vi "getState.vi"(8 "error in (no error)":errorcluster, 11 "UntilIntensityReading in":refnum<class "UntilIntensityReading.lvclass">) -> (0 "error out":errorcluster, 2 "StateValue":T1=enum."UntilIntensityReadingState", 3 "UntilIntensityReading out":refnum<class "UntilIntensityReading.lvclass">)   [LabVIEW 2016, in "UntilIntensityReading.lvclass"]
uses:
  UntilIntensityReading.lvclass
  ts_electrometeruserevents/Typedefs/StateValue.ctl
  ts_electrometeruserevents/Typedefs/ElectrometerTypedefs.lvlib
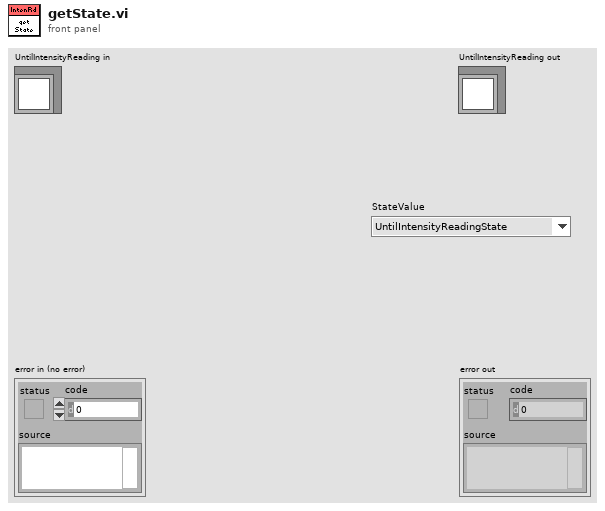
[diagram p1: front panel]
types:
  T1 = typedef "ElectrometerTypedefs.lvlib/StateValue.ctl" = enum16{"", "DisabledState", "EnabledState", "FaultState", "OffState", "StandbyState", "ReadyState", "ConfiguringState", "ManualReadingState", "UntilIntensityReadingState", "SetDurationReadingState", "BufferReadingState"}
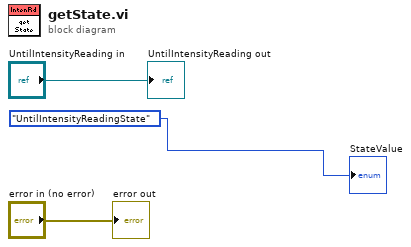
[diagram p0: block diagram]
diagram:
  "error out" <- "error in (no error)"
  "UntilIntensityReading out" <- "UntilIntensityReading in"
  "StateValue" <- StateValue."UntilIntensityReadingState" ("StateValue")
